vi "ArchiveLogsKiller.vi"   [LabVIEW 2011]
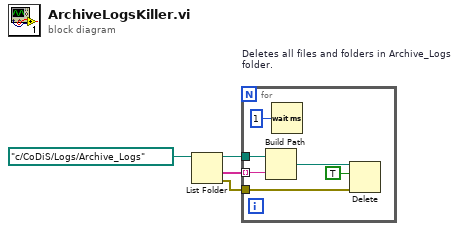
[diagram p0: block diagram]
diagram:
  w2 = path "c:/CoDiS/Logs/Archive_Logs"  # Deletes all files and folders in Archive_Logs folder.
  n1 = List Folder(path=w2) -> (path out=w1:path, folder names=w4:string[], error out=w3:errorcluster)  [unwired: 3 in, 1 out]
  n2 = for {
    tunnel: w4 -> [w9] mode=indexing
    tunnel: w3 -> [w5]
    tunnel: w1 -> [w10]
    n3 = Build Path(base path=w10, name or relative path=w9) -> (appended path=w7:path)
    n4 = Wait (ms)(milliseconds to wait=u32 1) -> ()  [unwired: 1 out]
    n5 = Delete(path (use dialog)=w7, entire hierarchy (F)=TRUE, error in=w5) -> ()  [unwired: 2 in, 3 out]
  }
